vi "_Read (No Objects) - LCD.vi"(8 "errorIN":errorcluster caption="Error", 11 "Cluster In":T1) -> (0 "errorOUT":errorcluster caption="Error out", 2 "X array":dbl[](array[numeric]), 3 "Cluster Out":T1)   [LabVIEW 2015]
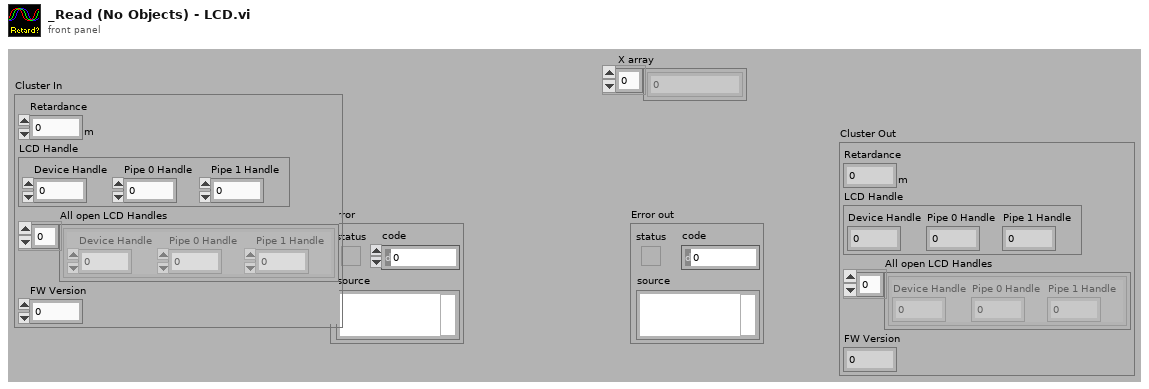
[diagram p1: front panel]
types:
  T1 = cluster{"Retardance":dbl[unit], "LCD Handle":cluster{"Device Handle":u32, "Pipe 0 Handle":u32, "Pipe 1 Handle":u32}, "All open LCD Handles":cluster{"Device Handle":u32, "Pipe 0 Handle":u32, "Pipe 1 Handle":u32}[], "FW Version":dbl}
  T2 = cluster{"Device Handle":u32, "Pipe 0 Handle":u32, "Pipe 1 Handle":u32}
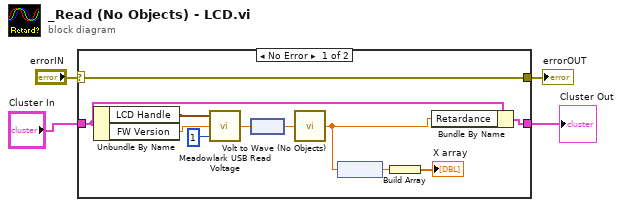
[diagram p0: block diagram]
diagram:
  n1 = case shown="No Error" "errorIN" {
    selector: "errorIN" -> [w9 w16]
    tunnel: [w15 w17] -> w1
    tunnel: "Cluster In" -> [w14 w17]
    tunnel: [w9 w16] -> w3
    frame No Error {
      n2 = Unbundle By Name(w14) -> ("LCD Handle"=w12:T2, "FW Version"=w11:dbl)
      n3 = call "Meadowlark USB Read Voltage.VI"("LC Channel"=1, "FW Version"=w11, "USB Open Device Cluster"=w12) -> ("Readout \nVoltage"=w10:dbl)
      n4 = node(w10) -> (w7:dbl[unit])
      n5 = call "Volt to Wave (No Objects).vi"("Voltage"=w7) -> ("Retardance"=w5:dbl[unit])
      n6 = node(w5) -> (w6:dbl)
      n7 = Build Array(w6) -> (→"X array":dbl[])
      n8 = Bundle By Name(cluster=w14, "Retardance"=w5) -> (w15:T1)
    }
    frame Error {
    }
  }
  "errorOUT" <- w3
  "Cluster Out" <- w1
